vi "Initialise.vi"(8 "error in (no error)":errorcluster, 9 "Buffer Size":i32=10, 11 "Dell Webcam in":refnum<class "Webcam.lvclass">) -> (0 "error out":errorcluster, 3 "Dell Webcam out":refnum<class "Webcam.lvclass">)   [LabVIEW 2019, in "Webcam.lvclass"]
uses:
  Webcam.lvclass
  <vilib>/vision/driver/IMAQdx.llb/IMAQdx Acquisition Mode.ctl
  Webcam.lvclass/Webcam.ctl
  <vilib>/vision/driver/NI_Vision_Acquisition_Software.lvlib
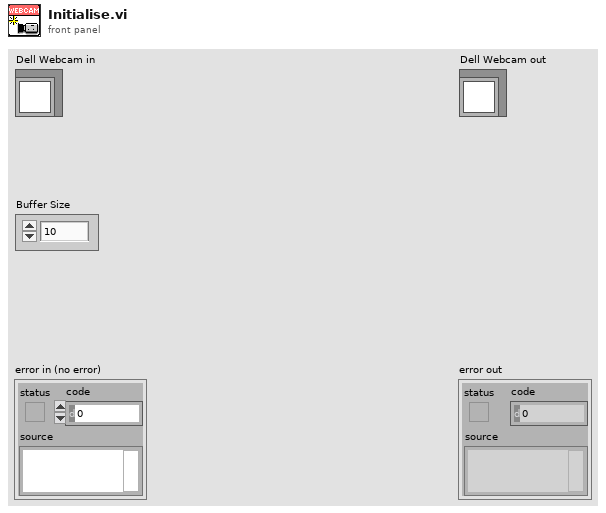
[diagram p1: front panel]
types:
  T1 = typedef "NI_Vision_Acquisition_Software.lvlib/IMAQdx Acquisition Mode.ctl" = enum32{"One Shot", "Continuous"}
  T2 = typedef "IMAQdx.ctl" = refnum<k21>
  T3 = typedef "Image Type" = u32
  T4 = typedef "IMAQ Image.ctl" = refnum<image>
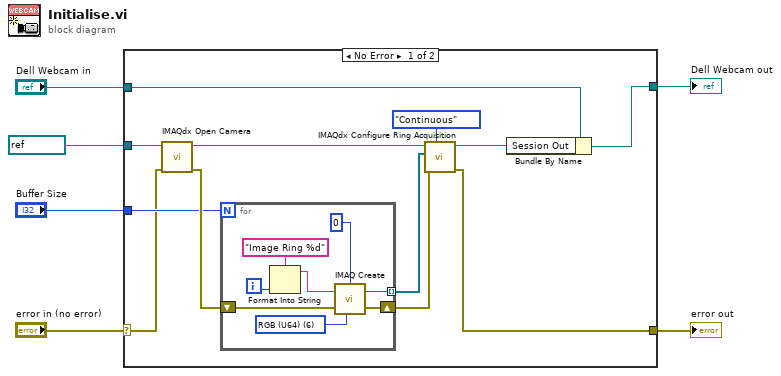
[diagram p0: block diagram]
diagram:
  n1 = case shown="No Error" "error in (no error)" {
    selector: "error in (no error)" -> [w7 w28]
    tunnel: refnum<k21> "cam0" ("Camera Name") -> [w14 _]
    tunnel: "Dell Webcam in" -> [w13 w27]
    tunnel: [w11 w27] -> w4
    tunnel: [w9 w28] -> w3
    tunnel: "Buffer Size" -> [w8 _]
    frame No Error {
      n2 = call <vilib>:"IMAQdx Open Camera.vi"("error in"=w7, "Session In"=w14) -> ("error out"=w16:errorcluster, "Session Out"=w18:T2)  [unwired: 1 in, 7 out]
      n3 = for {
        N: w8 -> [_]
        tunnel: [w25] -> w15 mode=indexing
        shift-right: [w24] -> w10
        shift-left: w16 -> [w26]
        i -> [w23]
        w19 = T3 6 items=["Grayscale (U8)", "Grayscale (I16)", "Grayscale (SGL)", "Complex (CSG)", "RGB (U32)", "HSL (U32)", "RGB (U64)", "Grayscale (U16)"] ("Image Type")
        n4 = Format Into String(format string="Image Ring %d" ("Image Name"), w23) -> (resulting string=w22:string)  [unwired: 2 in, 1 out]
        n5 = call "IMAQ Create"("Border Size"=0, "Image Name"=w22, "Image Type"=w19, "error in (no error)"=w26) -> ("New Image"=w25:T4, "error out"=w24:errorcluster)  [unwired: 1 out]
      }
      n6 = call <vilib>:"IMAQdx Configure Ring Acquisition.vi"("Mode"=IMAQdx_Acquisition_Mode."Continuous" ("Continuous?"), "error in"=w10, "Images"=w15, "Session In"=w18) -> ("error out"=w9:errorcluster, "Session Out"=w12:T2)  [unwired: 5 in, 1 out]
      n7 = Bundle By Name(cluster=w13, "Session Out"=w12) -> (w11:refnum<class "Webcam.lvclass">)
    }
    frame Error {
    }
  }
  "error out" <- w3
  "Dell Webcam out" <- w4
